vi "niFpga wdp fft pfft 2.vi"(6 "enable":bool, 11 "data in":T1(array[cluster])=[{"data re"=0.0, "data im"=0.0}, {"data re"=0.0, "data im"=0.0}]) -> (3 "data out":T2(array[cluster]))   [LabVIEW 2017]
types:
  T1 = cluster{"data re":fxp<+/-,8,1>, "data im":fxp<+/-,8,1>}[]
  T2 = cluster{"data re":fxp<+/-,8,1>, "data re":fxp<+/-,8,1>}[]
  T3 = cluster{"data re":fxp<+/-,8,1>, "data im":fxp<+/-,8,1>}
  T4 = cluster{"data re":fxp<+/-,8,1>, "data re":fxp<+/-,8,1>}
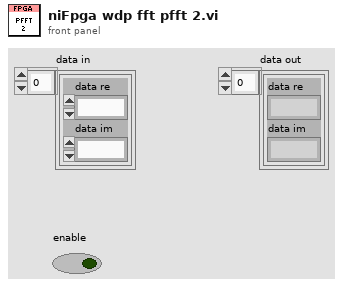
[diagram p1: front panel]
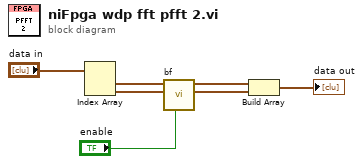
[diagram p0: block diagram]
diagram:
  n1 = Index Array(array="data in") -> (element #1=w2:T3, element #2=w3:T3)  [unwired: 2 in]
  n2 = call "bf"("enable"="enable", "data in 1"=w3, "data in 0"=w2) -> ("data out 1"=w6:T4, "data out 0"=w5:T4)  [unwired: 7 in]
  n3 = Build Array(w5, w6) -> (→"data out":T2)
